vi "library_variable.vi"() -> ()   [LabVIEW 2020, in "main.lvlib" / "stopwatch_timer.lvlib"]
uses:
  stopwatch_timer.lvlib
  stopwatch data.ctl
  state.ctl
panel:
  in  "stopwatch data":T1={"state"=enum."running", "started at"=timestamp(0 s since 1904-01-01), "last resumed at"=timestamp(0 s since 1904-01-01), "last paused at"=timestamp(0 s since 1904-01-01), "total time running (seconds)"=0.0, "total time paused (seconds)"=0.0} {"total time paused (seconds)" format="%.3f"; "total time running (seconds)" format="%.3f"}
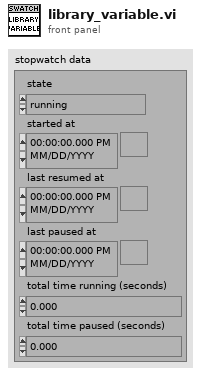
[diagram p1: front panel]
types:
  T1 = typedef "main.lvlib/stopwatch_timer.lvlib/stopwatch data.ctl" = cluster{"state":T2, "started at":timestamp, "last resumed at":timestamp, "last paused at":timestamp, "total time running (seconds)":dbl, "total time paused (seconds)":dbl}
  T2 = typedef "main.lvlib/stopwatch_timer.lvlib/state.ctl" = enum16{"not started", "running", "paused"}
diagram:
